vi "Update Message Getter.vi"(7 "RPC Message Name":string, 8 "error in (no error)":errorcluster, 10 "Message Getter in":refnum<vi>, 11 "RPC Messages Folder (ProjectItem) in":refnum<vi>) -> (0 "error out":errorcluster, 2 "Message Getter out":refnum<vi>, 3 "RPC Messages Folder (ProjectItem) out":refnum<vi>)   [LabVIEW 2019, in "gRPC Scripting Tools.lvlib"]
uses:
  gRPC Scripting Tools.lvlib
  <vilib>/Utility/traverseref.llb/VI Scripting - Traverse.lvlib
  <vilib>/Utility/traverseref.llb/TRef TravTarget.ctl
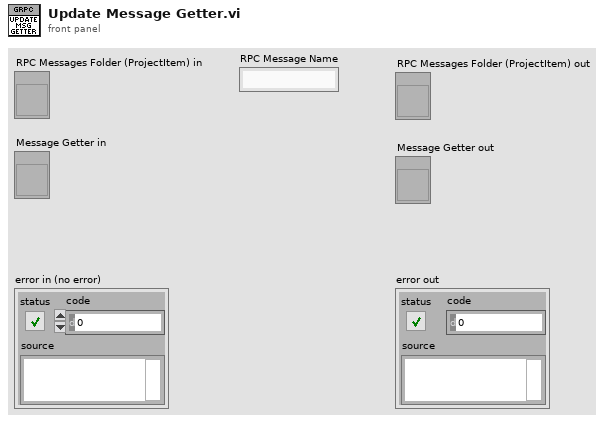
[diagram p1: front panel]
types:
  T1 = typedef "TRef TravTarget.ctl" = enum16{"FP", "BD", "Other"}
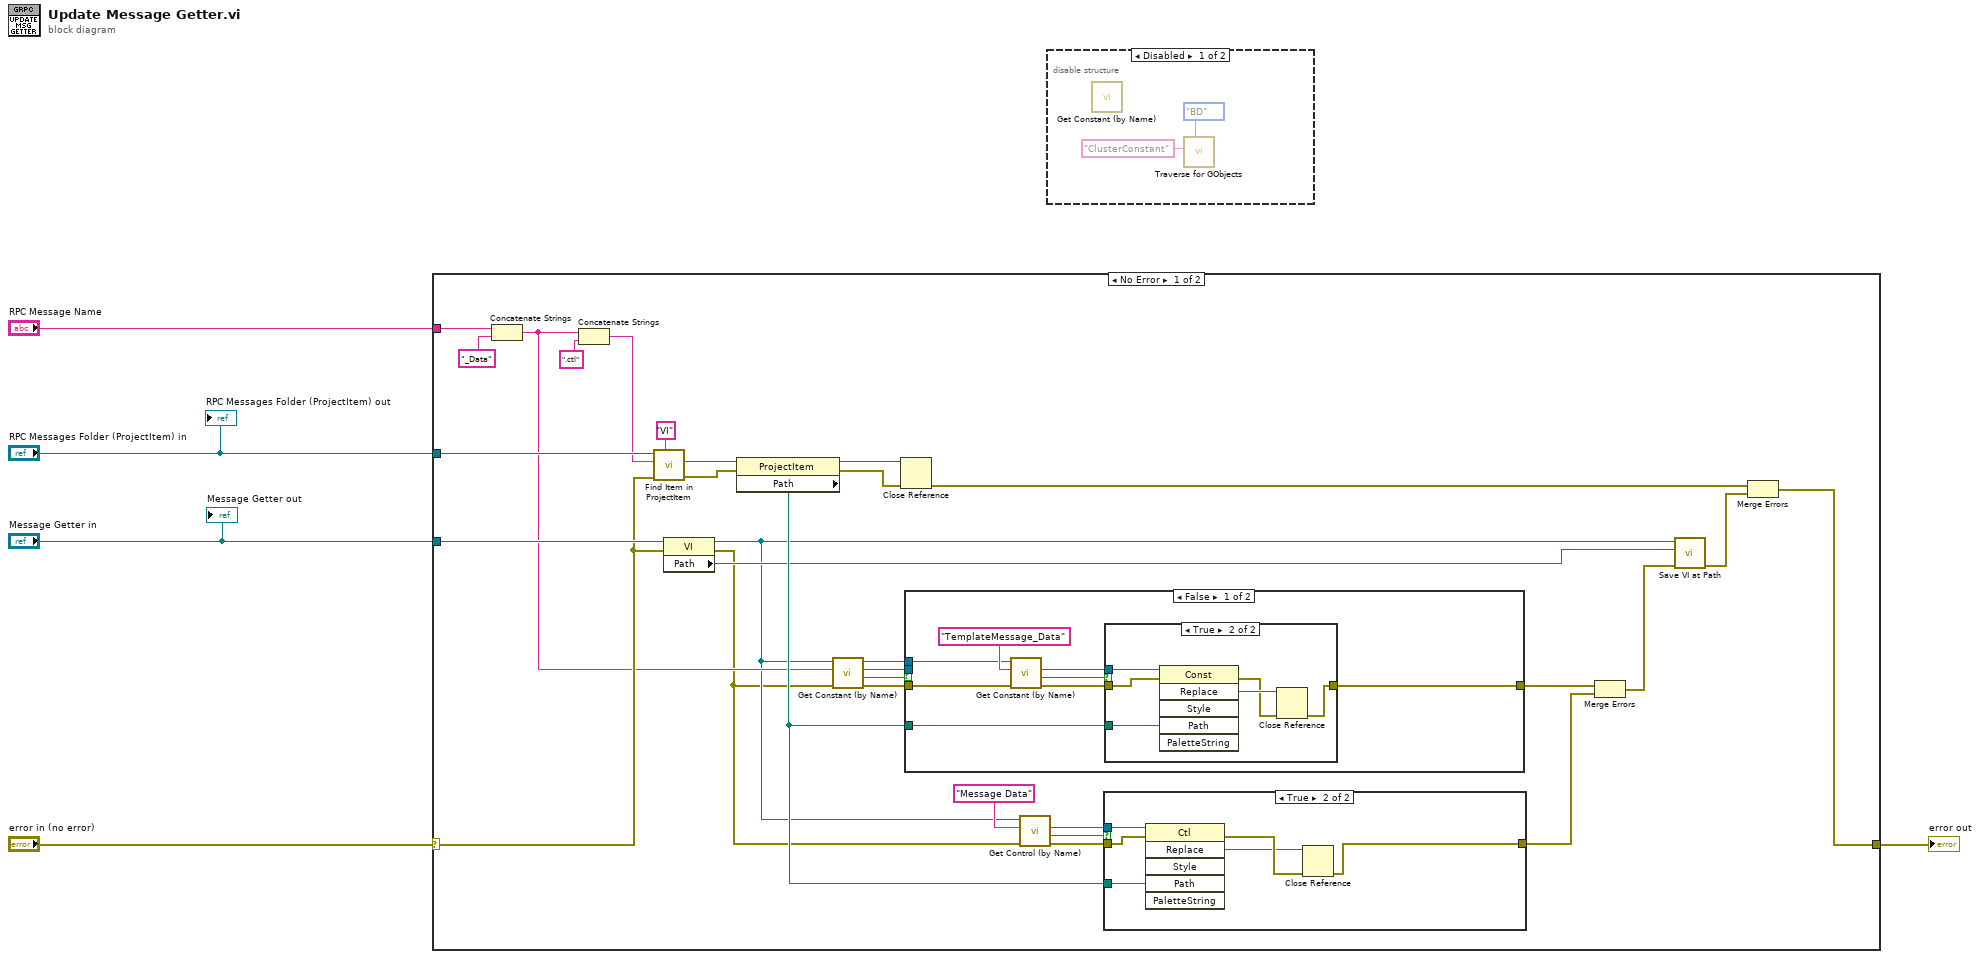
[diagram p0: block diagram]
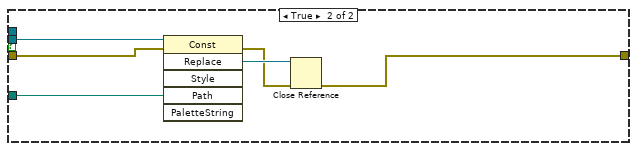
[diagram p4: hidden frame]
diagram:
  n1 = case shown="No Error" "error in (no error)" {
    selector: "error in (no error)" -> [w19 w65]
    tunnel: "Message Getter in" -> [w31 _]
    tunnel: [w30 w65] -> w4
    tunnel: "RPC Message Name" -> [w22 _]
    tunnel: "RPC Messages Folder (ProjectItem) in" -> [w20 _]
    frame No Error {
      n2 = Concatenate Strings(w22, "_Data" ("string")) -> (w10:string)
      n3 = Concatenate Strings(w10, ".ctl" ("string")) -> (w14:string)
      n4 = call "Find Item in ProjectItem.vi"("Item Type"="VI", "error in (no error)"=w19, "Name"=w14, "ProjectItem in"=w20) -> ("error out"=w25:errorcluster, "Item Refnum out"=w24:refnum<vi>)  [unwired: 4 in, 2 out]
      n5 = property class="VI"(reference=w31, error in=w19) -> (reference out=w9:refnum<vi>, error out=w8:errorcluster, "Path"=w32:path)
      n6 = property class="ProjectItem"(reference=w24, error in=w25) -> (reference out=w26:refnum<vi>, error out=w27:errorcluster, "Path"=w33:path)
      n7 = call "Get Constant (by Name).vi"("error in (no error)"=w8, "Constant Label"=w10, "Owner VI in"=w9) -> ("error out"=w12:errorcluster, "Found ?"=w7:bool, "Const ref out"=w6:refnum<vi>, "Owner VI out"=w11:refnum<vi>)  [unwired: 5 in]
      n8 = Close Reference(reference=w26, error in (no error)=w27) -> (error out=w29:errorcluster)
      n9 = case shown="False" w7 {
        tunnel: [w44 w52] -> w34
        tunnel: w33 -> [w43 w53]
        tunnel: w12 -> [w38 w57]
        tunnel: w11 -> [w37 _]
        tunnel: w6 -> [_ w56]
        frame False {
          n10 = call "Get Constant (by Name).vi"("error in (no error)"=w38, "Constant Label"="TemplateMessage_Data" ("name/order"), "Owner VI in"=w37) -> ("error out"=w40:errorcluster, "Found ?"=w39:bool, "Const ref out"=w42:refnum<vi>)  [unwired: 5 in, 1 out]
          n11 = case shown="True" w39 {
            tunnel: [w45 w51] -> w44
            tunnel: w43 -> [_ w50]
            tunnel: w42 -> [_ w47]
            tunnel: w40 -> [w45 w46]
            frame False {
            }
            frame True {
              n12 = invoke class="Const" method="Replace"(reference=w47, error in=w46, "Path"=w50) -> (error out=w48:errorcluster, "Replace"=w49:refnum<vi>)  [unwired: 3 in, 4 out]
              n13 = Close Reference(reference=w49, error in (no error)=w48) -> (error out=w51:errorcluster)
            }
          }
        }
        frame True {
          n14 = invoke class="Const" method="Replace"(reference=w56, error in=w57, "Path"=w53) -> (error out=w54:errorcluster, "Replace"=w55:refnum<vi>)  [unwired: 3 in, 4 out]
          n15 = Close Reference(reference=w55, error in (no error)=w54) -> (error out=w52:errorcluster)
        }
      }
      n16 = call "Get Control (by Name).vi"("error in (no error)"=w8, "Control Label"="Message Data" ("name/order"), "Owner VI in"=w9) -> ("error out"=w16:errorcluster, "Found ?"=w13:bool, "Control Refnum"=w17:refnum<vi>)  [unwired: 5 in, 1 out]
      n17 = case shown="True" w13 {
        tunnel: [w58 w64] -> w35
        tunnel: w33 -> [_ w61]
        tunnel: w17 -> [_ w60]
        tunnel: w16 -> [w58 w59]
        frame False {
        }
        frame True {
          n18 = invoke class="Ctl" method="Replace"(reference=w60, error in=w59, "Path"=w61) -> (error out=w63:errorcluster, "Replace"=w62:refnum<vi>)  [unwired: 3 in, 4 out]
          n19 = Close Reference(reference=w62, error in (no error)=w63) -> (error out=w64:errorcluster)
        }
      }
      n20 = Merge Errors(w34, w35) -> (w36:errorcluster)
      n21 = call "Save VI at Path.vi"("error in (no error)"=w36, "Path"=w32, "VI in"=w9) -> ("error out"=w28:errorcluster)  [unwired: 6 in, 2 out]
      n22 = Merge Errors(w29, w28) -> (w30:errorcluster)
    }
    frame Error {
    }
  }
  "error out" <- w4
  n23 = disable-structure shown="Disabled" {
    frame Disabled {
      n24 = call "Get Constant (by Name).vi"() -> ()  [unwired: 8 in, 4 out]
      n25 = call <vilib>:"Traverse for GObjects.vi"("Traverse Target"=TRef_TravTarget."BD", "Class Name"="ClusterConstant") -> ()  [unwired: 6 in, 4 out]
    }
    frame Enabled {
    }
  }
  "RPC Messages Folder (ProjectItem) out" <- "RPC Messages Folder (ProjectItem) in"
  "Message Getter out" <- "Message Getter in"
